vi "Where_to_find_EV3.vi"   [LabVIEW 2012]
uses:
  SubVIs/LVPresent_Globals.vi
panel:
  # "Where to Find What?\n\nCheck out the pictures below to figure out where to open the Block and Front diagrams, and how to open the Controls Palette (Front diagram), Functions Palette (Block diagram), and Tools Palette (can be used for both)."
  # "Block Diagram"
  # "Front Diagram"
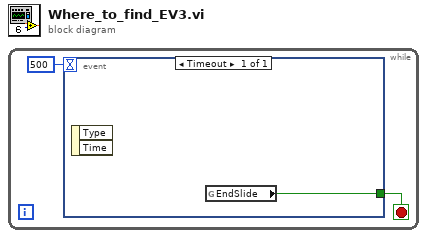
[diagram p0: block diagram]
diagram:
  n1 = while {
    stop <- w2 stop-if-true
    n2 = event shown="[0] Timeout" {
      selector: _ -> [_]
      dyn-events: _ -> [_]
      timeout: 500 -> [_]
      tunnel: [w3] -> w2
      event Timeout {
        n3 = event-data() -> ()  [unwired: 1 in, 2 out]
        n4 = global read "LVPresent_Globals.vi" "EndSlide"() -> (w3:bool)
      }
    }
  }
